vi "GetPlotReference.vi"(8 "error in":errorcluster, 11 "Plot in":refnum<class "Plot.lvclass">) -> (0 "error out":errorcluster, 1 "plot reference":refnum<vi>, 3 "Plot out":refnum<class "Plot.lvclass">)   [LabVIEW 2014, in "Plot.lvclass"]
uses:
  Plot.lvclass
  Plot.lvclass/Plot.ctl
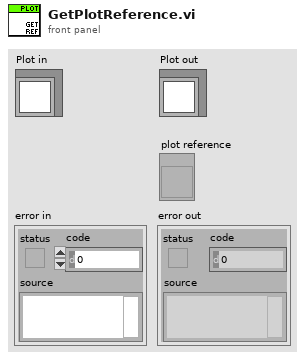
[diagram p1: front panel]
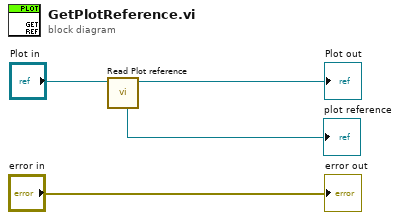
[diagram p0: block diagram]
diagram:
  n1 = call "Read Plot reference.vi"("Plot in"="Plot in") -> ("Plot out"=→"Plot out":refnum<class "Plot.lvclass">, "Plot reference"=→"plot reference":refnum<vi>)  [unwired: 7 in]
  "error out" <- "error in"
